vi "AIT 1553 - Create BM Sysdef Tree Messages.vi"(7 "Called From SysDef API (F)":bool, 8 "error in":errorcluster, 9 "BM Messages":T1[](array[typedef]), 10 "Section Ptr":T3 format="%.0x") -> (0 "error out":errorcluster)   [LabVIEW 2013]
uses:
  <vilib>/NI Veristand/Custom Device API/Custom Device Item Ref.ctl
  Controls/1553_BM_Message.ctl
  Controls/664 -Param.ctl
  <vilib>/NI Veristand/Custom Device API/Custom Device Channel Type.ctl
  <vilib>/NI Veristand/Custom Device API/Custom Device Channel.ctl
  Controls and Global/Global.vi
  <vilib>/NI Veristand/Custom Device API/Custom Device API.lvlib
  AIT 664 Custom Device.lvlib
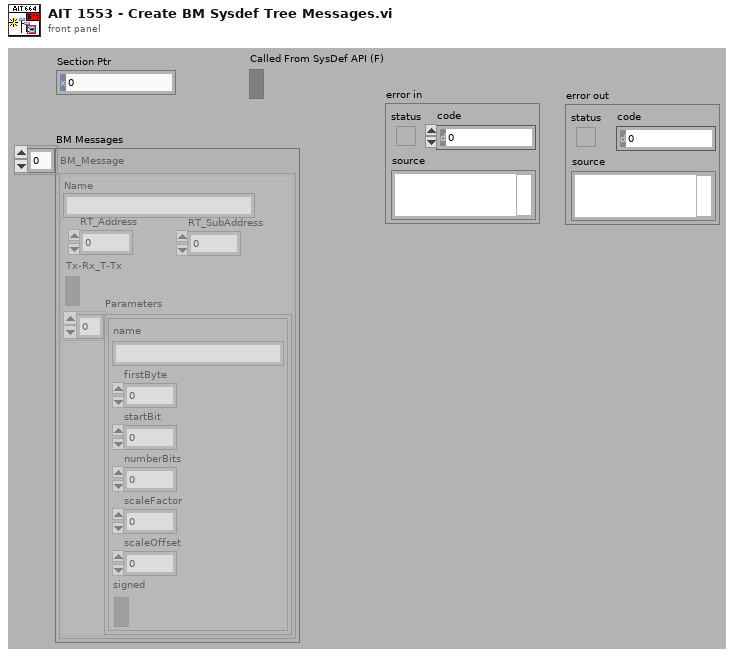
[diagram p1: front panel]
types:
  T1 = typedef "AIT 664 Custom Device.lvlib/1553_BM_Message.ctl" = cluster{"RT_Address":u8, "RT_SubAddress":u8, "Tx-Rx_T-Tx":bool, "Parameters":T2[], "Name":string}
  T2 = typedef "AIT 664 Custom Device.lvlib/664 -Param.ctl" = cluster{"name":string, "firstByte":i32, "startBit":i32, "numberBits":i32, "scaleFactor":dbl, "scaleOffset":dbl, "signed":bool}
  T3 = typedef "Custom Device API.lvlib/Custom Device Item Ref.ctl" = u64
  T4 = typedef "Custom Device API.lvlib/Custom Device Channel.ctl" = cluster{"Type":T5, "Units":string, "Default Value":dbl, "Faultable":bool, "Scalable":bool}
  T5 = typedef "Custom Device API.lvlib/Custom Device Channel Type.ctl" = enum16{"Input", "Output"}
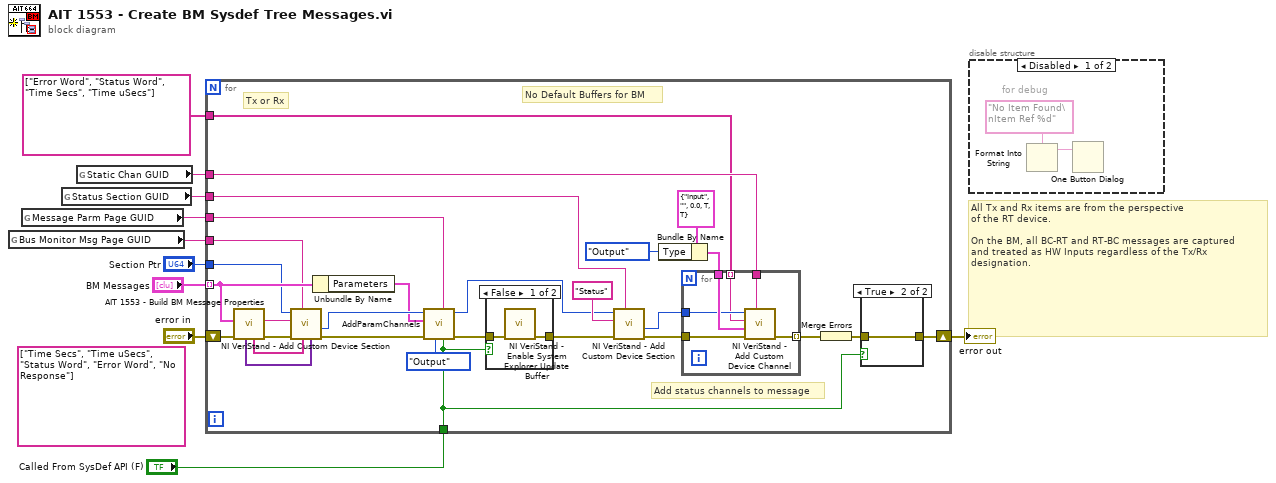
[diagram p0: block diagram]
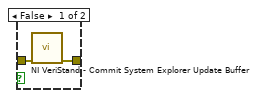
[diagram p3: hidden frame]
diagram:
  (unwired) string[] ["Time Secs", "Time uSecs", "Status Word", "Error Word", "No Response"]
  # "All Tx and Rx items are from the perspective \nof the RT device.\n\nOn the BM, all BC-RT and RT-BC messages are captured\nand treated as HW Inputs regardless of the Tx/Rx \ndesignation."
  n1 = global read "Global.vi" "Bus Monitor Msg Page GUID"() -> (w7:string)
  n2 = global read "Global.vi" "Message Parm Page GUID"() -> (w5:string)
  n3 = global read "Global.vi" "Status Section GUID"() -> (w3:string)
  n4 = global read "Global.vi" "Static Chan GUID"() -> (w4:string)
  n5 = for {
    shift-right: [w12] -> w10
    shift-left: "error in" -> [w35]
    tunnel: "Section Ptr" -> [w30]
    tunnel: "BM Messages" -> [w32] mode=indexing
    tunnel: w7 -> [w31]
    tunnel: w5 -> [w29]
    tunnel: w4 -> [w27]
    tunnel: w3 -> [w17]
    tunnel: string[] ["Error Word", "Status Word", "Time Secs", "Time uSecs"] -> [w26]
    tunnel: "Called From SysDef API (F)" -> [w11]
    # "Add status channels to message"
    # "Tx or Rx"
    # "No Default Buffers for BM"
    n6 = call "AIT 1553 - Build BM Message Properties.vi"("error in (no error)"=w35, "BM_Message"=w32) -> ("error out"=w37:errorcluster, "name"=w36:string, "Prop Names"=w38:string[], "Prop Values"=w39:variant[])  [unwired: 5 in, 1 out]
    n7 = call <vilib>:"NI VeriStand - Add Custom Device Section.vi"("Property Values"=w39, "Property names"=w38, "GUID (Default Section)"=w31, "error in (no error)"=w37, "Section Name"=w36, "Parent Ref in"=w30) -> ("error out"=w33:errorcluster, "Section Ptr"=w34:T3)  [unwired: 2 in, 2 out]
    n8 = Unbundle By Name(w32) -> ("Parameters"=w25:T2[])
    n9 = call "AddParamChannels.vi"("Called From SysDef API (F)"=w11, "Parm Page GUID"=w29, "Type"=Custom_Device_Channel_Type."Output", "error in"=w33, "Parameters to add"=w25, "Node Ref In"=w34) -> ("error out"=w15:errorcluster, "Node Ref Out"=w16:T3)  [unwired: 4 in]
    n10 = case shown="False" w11 {
      tunnel: w15 -> [w44 w45]
      tunnel: [w43 w45] -> w14
      frame False {
        n11 = call <vilib>:"NI VeriStand - Enable System Explorer Update Buffer.vi"("error in (no error)"=w44) -> ("error out"=w43:errorcluster)  [unwired: 10 in]
      }
      frame True {
      }
    }
    n12 = call <vilib>:"NI VeriStand - Add Custom Device Section.vi"("GUID (Default Section)"=w17, "error in (no error)"=w14, "Section Name"="Status", "Parent Ref in"=w16) -> ("error out"=w22:errorcluster, "Section Ptr"=w23:T3)  [unwired: 4 in, 2 out]
    n13 = Bundle By Name(cluster=T4 {"Type"=enum."Input", "Units"="", "Default Value"=0.0, "Faultable"=TRUE, "Scalable"=TRUE} ("Channel"), "Type"=Custom_Device_Channel_Type."Output") -> (w21:T4)
    n14 = for {
      tunnel: [w51] -> w18 mode=indexing
      tunnel: w21 -> [w50]
      tunnel: w27 -> [w49]
      tunnel: w22 -> [w48]
      tunnel: w23 -> [w47]
      tunnel: w26 -> [w46] mode=indexing
      n15 = call <vilib>:"NI VeriStand - Add Custom Device Channel.vi"("GUID (Default Channel)"=w49, "error in (no error)"=w48, "Channel"=w50, "Channel Name"=w46, "Parent Ref in"=w47) -> ("error out"=w51:errorcluster)  [unwired: 3 in, 3 out]
    }
    n16 = Merge Errors(w18) -> (w13:errorcluster)
    n17 = case shown="True" w11 {
      tunnel: w13 -> [w41 w42]
      tunnel: [w40 w42] -> w12
      frame False {
        n18 = call <vilib>:"NI VeriStand - Commit System Explorer Update Buffer.vi"("error in (no error)"=w41) -> ("error out"=w40:errorcluster)  [unwired: 10 in]
      }
      frame True {
      }
    }
  }
  "error out" <- w10
  n19 = disable-structure shown="Disabled" {
    frame Disabled {
      # "for debug"
      n20 = Format Into String(format string="No Item Found\nItem Ref %d" ("message")) -> (resulting string=w54:string, w52:T3)  [unwired: 2 in, 1 out]
      n21 = One Button Dialog(message=w54) -> (true=w55:bool)  [unwired: 1 in]
    }
    frame Enabled {
    }
  }
